vi "Read.vi"   [LabVIEW 2020, in "Agilent 3446X Series.lvlib"]
doc: "Allows users to read one or more measurements from the DMM."
uses:
  Agilent 3446X Series.lvlib
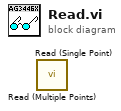
[diagram p0: block diagram]
diagram:
  n1 = call "Read (Multiple Points).vi"() -> ()  [unwired: 9 in, 3 out]
  n2 = call "Read (Single Point).vi"() -> ()  [unwired: 9 in, 3 out]
